vi "DisableCtrls.vi"(10 "Array":refnum<vi>[](array[refnum]), 11 "Enabled?":bool) -> ()   [LabVIEW 2021]
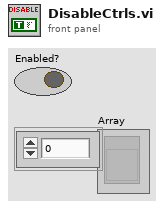
[diagram p1: front panel]
types:
  T1 = enum8{"Enabled", "Disabled", "Disabled and Grayed Out"}
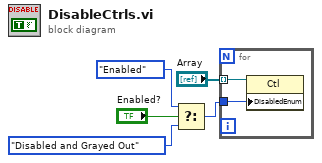
[diagram p0: block diagram]
diagram:
  n1 = Select(t=T1."Enabled", s="Enabled?", f=T1."Disabled and Grayed Out" ("Disabled")) -> (s? t:f=w4:T1)
  n2 = for {
    tunnel: w4 -> [w7]
    tunnel: "Array" -> [w6] mode=indexing
    n3 = property on="Property Node" class="Ctl"(reference=w6, "DisabledEnum"=w7) -> ()  [unwired: 1 in, 2 out]
  }
